vi "Encoder Turn.vi"(10 "Setpoint":dbl=-4.0 format="%.2f", 11 "Execute?":bool) -> (3 "Done":bool)   [LabVIEW 2012]
uses:
  Globals/Useful Values.vi
  <vilib>/addons/control/pid/pid.llb/PID (DBL).vi
  <vilib>/addons/control/pid/NI_PID_pid.lvlib
panel:
  out "Turn":dbl=-0.09989639700515257
  in  "PID gains":T1={"proportional gain (Kc)"=0.23, "integral time (Ti, min)"=0.0, "derivative time (Td, min)"=0.0}
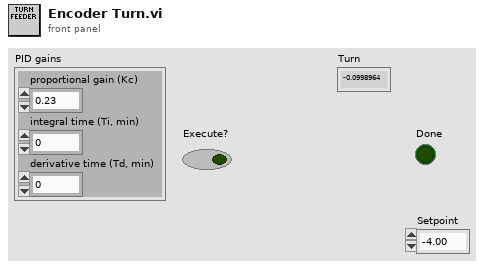
[diagram p1: front panel]
types:
  T1 = cluster{"proportional gain (Kc)":dbl, "integral time (Ti, min)":dbl, "derivative time (Td, min)":dbl}
  T2 = typedef "WPI_GyroDevRef.ctl" = cluster{"DevStatus":errorcluster, "Analog Module":T3, "Analog Channel":T4, "Offset":dbl, "Gain (VoltsPerDegree/Second)":dbl}
  T3 = typedef "FPGA_TypedefAnalogModule.ctl" = enum16{"Analog Module 1", "Analog Module 2"}
  T4 = typedef "FPGA_AIChannel.ctl" = enum8{"AI 1", "AI 2", "AI 3", "AI 4", "AI 5", "AI 6", "AI 7", "AI 8", "Invalid"}
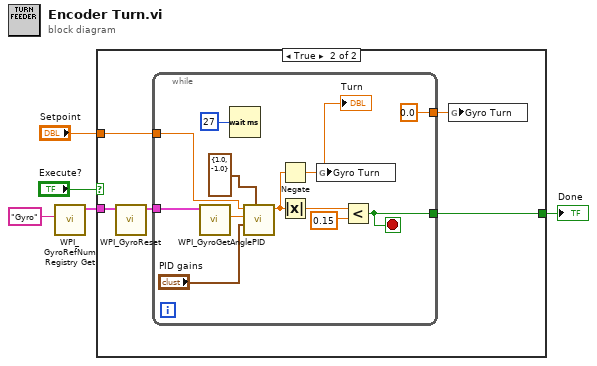
[diagram p0: block diagram]
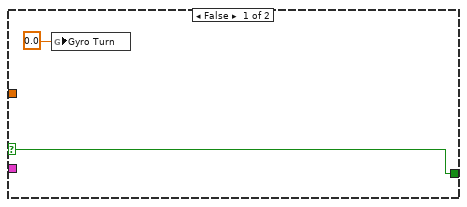
[diagram p2: hidden frame]
diagram:
  n1 = call <vilib>:"WPI_GyroRefNum Registry Get.vi"("refnum name"="Gyro") -> ("GyroDevRef"=w1:T2)  [unwired: 9 in, 1 out]
  n2 = case shown="True" "Execute?" {
    selector: "Execute?" -> [w7 _]
    tunnel: [w7 w11] -> w4
    tunnel: "Setpoint" -> [_ w12]
    tunnel: w1 -> [_ w9]
    frame False {
      n3 = global write "Useful Values.vi" "Gyro Turn"(0.0 ("Encoder PID")) -> ()
    }
    frame True {
      n4 = call <vilib>:"WPI_GyroReset.vi"("GyroDevRef"=w9) -> ("GyroDevRef"=w8:T2)  [unwired: 9 in, 1 out]
      n5 = while {
        tunnel: w12 -> [w23]
        tunnel: [w19] -> w11
        tunnel: [0.0 ("Encoder PID")] -> w10
        tunnel: w8 -> [w17]
        stop <- w19 stop-if-true
        n6 = call <vilib>:"WPI_GyroGetAngle.vi"("GyroDevRef"=w17) -> ("Angle"=w16:dbl)  [unwired: 7 in, 3 out]
        n7 = Wait (ms)(milliseconds to wait=u32 27) -> ()  [unwired: 1 out]
        n8 = call-poly <vilib>:"PID.vi"("output range"=cluster{"output high":dbl, "output low":dbl} {"output high"=1.0, "output low"=-1.0}, "PID gains"="PID gains", "process variable"=w16, "setpoint"=w23) -> ("output"=w21:dbl)  [unwired: 6 in, 1 out]
        n9 = Negate(x=w21) -> (-x=w14:dbl)
        "Turn" <- w14
        n10 = Absolute Value(x=w21) -> (abs(x)=w22:dbl)
        n11 = global write "Useful Values.vi" "Gyro Turn"(w14) -> ()
        n12 = Less?(x=w22, y=0.15) -> (x < y?=w19:bool)
      }
      n13 = global write "Useful Values.vi" "Gyro Turn"(w10) -> ()
    }
  }
  "Done" <- w4
